vi "serial communication (licor).vi"(4 "time (global)":dbl, 5 "Fehler":errorcluster caption="error in", 6 "command":string, 7 "read buffer in":string, 8 "VISA resource":refnum<visa-resource-name>) -> (0 "Fehler (Ausgang)":errorcluster caption="error out", 1 "Licor-output":T1[](array[typedef]) {"time (global)" format="%<%H:%M:%S\n%d/%m/%Y>T"}, 2 "read buffer out":string, 3 "VISA resource out":refnum<visa-resource-name>)   [LabVIEW 2010, in "Licor-Steuerung.lvlib"]
uses:
  Licor-Steuerung.lvlib
  LicorLI7000/conventions/output line.ctl
  control/Emulate Licor output GV.vi
  LicorLI7000/LicorLI7000.lvlib
panel:
  out "Numerisch":i32
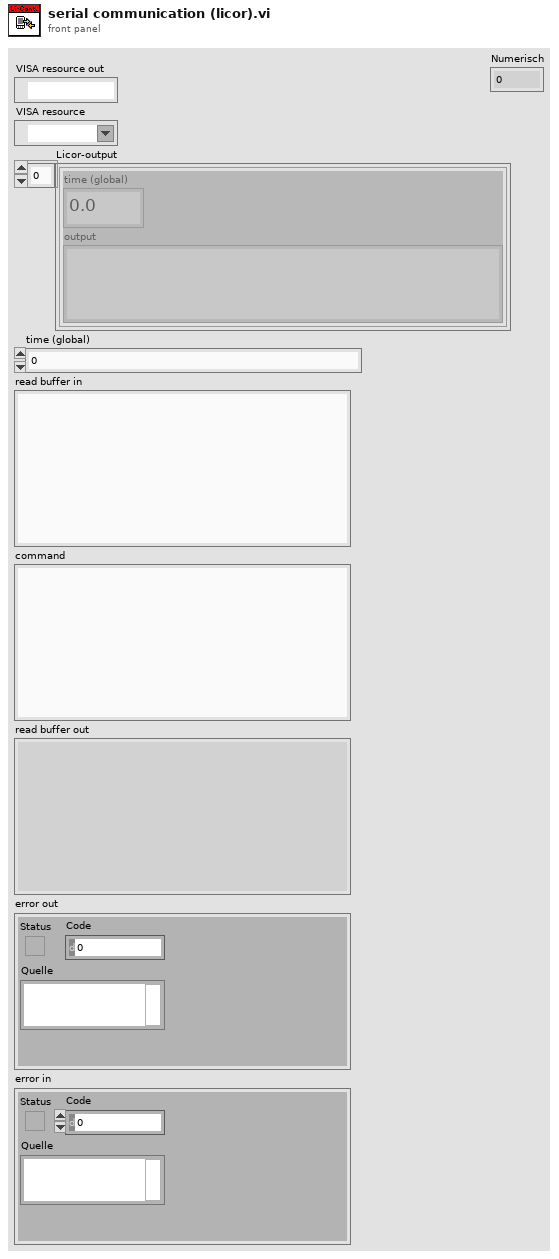
[diagram p1: front panel]
types:
  T1 = typedef "LicorLI7000.lvlib/output line.ctl" = cluster{"time (global)":dbl, "output":string}
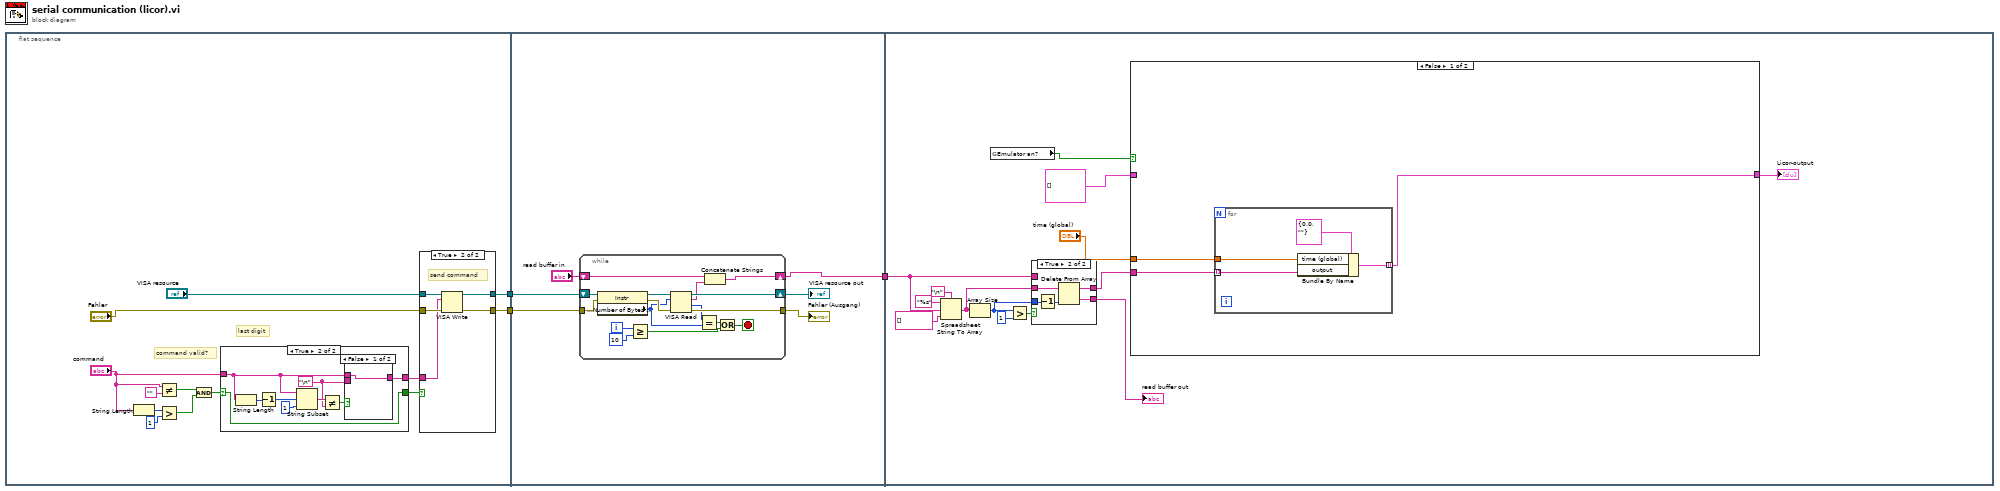
[diagram p0: block diagram]
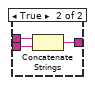
[diagram p4: hidden frame]
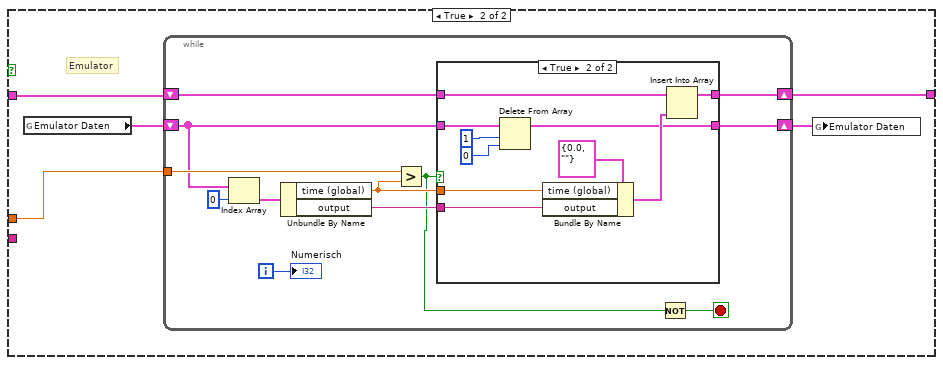
[diagram p5: hidden frame]
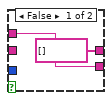
[diagram p7: hidden frame]
diagram:
  n1 = flat-sequence {
    tunnel: [w6] -> w2
    tunnel: [w5] -> w1
    tunnel: [w39] -> w3
    tunnel: w2 -> [w42]
    tunnel: w1 -> [w41]
    tunnel: w3 -> [w67]
    frame #0 {
      # "last digit"
      # "command valid?"
      n2 = String Length(string="command") -> (length=w9:i32)
      n3 = Not Equal?(x="command", y="") -> (x != y?=w8:bool)
      n4 = Greater?(x=w9, y=1) -> (0:w11:bool)
      n5 = Compound Arithmetic op=AND(w8, w11) -> (w12:bool)
      n6 = case shown="True" w12 {
        selector: w12 -> [w24 w27]
        tunnel: "command" -> [w25 w29]
        tunnel: [w25 w28] -> w16
        tunnel: [w24 w27] -> w14
        frame False {
        }
        frame True {
          w26 = "\n"
          n7 = String Length(string=w29) -> (length=w34:i32)
          n8 = Decrement(x=w34) -> (x-1=w33:i32)
          n9 = String Subset(string=w29, offset (0)=w33, length (rest)=1 ("Länge (Rest)")) -> (substring=w30:string)
          n10 = Not Equal?(x=w30, y=w26) -> (x != y?=w31:bool)
          n11 = case shown="False" w31 {
            tunnel: w29 -> [w35 w38]
            tunnel: w26 -> [_ w37]
            tunnel: [w35 w36] -> w28
            frame False {
            }
            frame True {
              n12 = Concatenate Strings(w38, w37) -> (w36:string)
            }
          }
        }
      }
      n13 = case shown="True" w14 {
        tunnel: "VISA resource" -> [w18 w23]
        tunnel: "Fehler" -> [w17 w22]
        tunnel: w16 -> [_ w21]
        tunnel: [w18 w20] -> w6
        tunnel: [w17 w19] -> w5
        frame False {
        }
        frame True {
          # "send command"
          n14 = VISA Write(VISA resource name=w23, write buffer=w21, error in (no error)=w22) -> (VISA resource name out=w20:refnum<visa-resource-name>, error out=w19:errorcluster)  [unwired: 1 out]
        }
      }
    }
    frame #1 {
      n15 = while {
        shift-right: [w60] -> w40
        shift-left: w42 -> [w50]
        tunnel: [w59] -> w43
        shift-right: [w58] -> w39
        shift-left: "read buffer in" -> [w57]
        tunnel: w41 -> [w47]
        i -> [w55]
        stop <- w51 stop-if-true
        n16 = property class="Instr"(reference=w50, error in=w47) -> (reference out=w49:refnum<visa-resource-name>, error out=w48:errorcluster, "Serial Settings:Number of Bytes at Serial Port"=w46:u32)
        n17 = Greater Or Equal?(x=w55, y=10) -> (x >= y?=w52:bool)
        n18 = VISA Read(VISA resource name=w49, byte count=w46, error in (no error)=w48) -> (VISA resource name out=w60:refnum<visa-resource-name>, read buffer=w45:string, return count=w56:u32, error out=w59:errorcluster)
        n19 = Equal?(x=w56, y=w46) -> (x = y?=w53:bool)
        n20 = Concatenate Strings(w57, w45) -> (w58:string)
        n21 = Or(x=w53, y=w52) -> (x .or. y?=w51:bool)
      }
      "Fehler (Ausgang)" <- w43
      "VISA resource out" <- w40
    }
    frame #2 {
      n22 = Spreadsheet String To Array(delimiter (Tab)="\n", format string="%s", spreadsheet string=w67, array type (2D Dbl)=string[] []) -> (array=w72:string[])
      n23 = Array Size(array=w72) -> (size(s)=w73:i32)
      n24 = global read "Emulate Licor output GV.vi" "Emulator an?"() -> (w62:bool)
      n25 = Greater?(x=w73, y=1) -> (0:w74:bool)
      n26 = case shown="True" w74 {
        tunnel: w73 -> [_ w116]
        tunnel: w72 -> [_ w115]
        tunnel: [w112 w114] -> w66
        tunnel: w67 -> [w112 _]
        tunnel: [string[] [] w113] -> w63
        frame False {
        }
        frame True {
          n27 = Decrement(x=w116) -> (x-1=w117:i32)
          n28 = Delete From Array(array=w115, index=w117) -> (deleted portion=w114:string, array with subset deleted=w113:string[])  [unwired: 1 in]
        }
      }
      "read buffer out" <- w66
      n29 = case shown="False" w62 {
        tunnel: "time (global)" -> [w77 w86]
        tunnel: [w75 w84] -> w64
        tunnel: w63 -> [w76 _]
        tunnel: T1[] [] -> [_ w85]
        frame False {
          n30 = for {
            tunnel: w76 -> [w80] mode=indexing
            tunnel: [w79] -> w75 mode=indexing
            tunnel: w77 -> [w78]
            n31 = Bundle By Name(cluster=T1 {"time (global)"=0.0, "output"=""} ("output line"), "time (global)"=w78, "output"=w80) -> (w79:T1)
          }
        }
        frame True {
          # "Emulator"
          n32 = global read "Emulate Licor output GV.vi" "Emulator Daten"() -> (w83:T1[])
          n33 = while {
            tunnel: w86 -> [w95]
            shift-right: [w92] -> w84
            shift-left: w85 -> [w91]
            shift-right: [w87] -> w82
            shift-left: w83 -> [w88]
            i -> [w93]
            stop <- w89 stop-if-true
            n34 = Index Array(array=w88, index=0 ("Index")) -> (element=w97:T1)
            n35 = Unbundle By Name(w97) -> ("time (global)"=w94:dbl, "output"=w96:string)
            n36 = Greater?(x=w95, y=w94) -> (0:w90:bool)
            n37 = case shown="True" w90 {
              tunnel: w88 -> [w99 w109]
              tunnel: w96 -> [_ w105]
              tunnel: w94 -> [_ w106]
              tunnel: [w100 w103] -> w92
              tunnel: w91 -> [w100 w102]
              tunnel: [w99 w101] -> w87
              frame False {
              }
              frame True {
                n38 = Delete From Array(array=w109, length=1 ("Länge"), index=0 ("Index")) -> (array with subset deleted=w101:T1[])  [unwired: 1 out]
                n39 = Bundle By Name(cluster=T1 {"time (global)"=0.0, "output"=""} ("output line"), "time (global)"=w106, "output"=w105) -> (w104:T1)
                n40 = Insert Into Array(array=w102, new element=w104) -> (w103:T1[])  [unwired: 1 in]
              }
            }
            n41 = Not(x=w90) -> (.not. x?=w89:bool)
            "Numerisch" <- w93
          }
          n42 = global write "Emulate Licor output GV.vi" "Emulator Daten"(w82) -> ()
        }
      }
      "Licor-output" <- w64
    }
  }
